vi "Matlab Param Array to Variant.vi"(8 "error in (no error)":errorcluster, 10 "Name":string, 11 "Variables":cluster{"Name":string, "Data":variant}[](array[cluster])) -> (0 "error out":errorcluster, 3 "Data":variant)   [LabVIEW 2010, in "Matlab API.lvlib"]
uses:
  Matlab API.lvlib
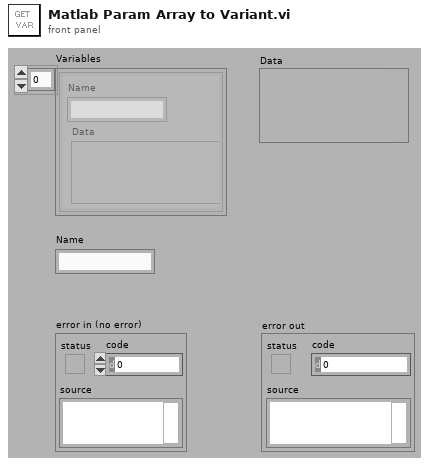
[diagram p1: front panel]
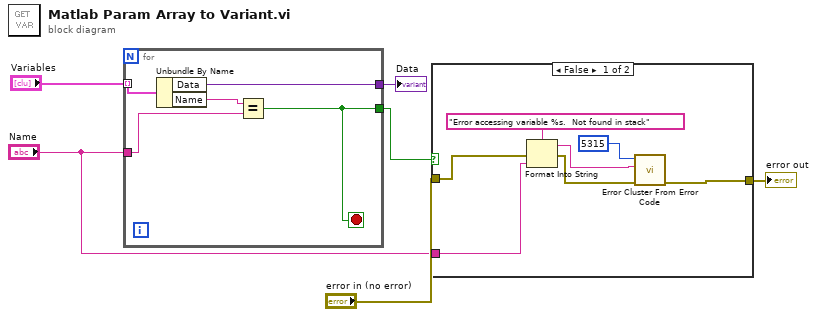
[diagram p0: block diagram]
diagram:
  n1 = for {
    tunnel: "Variables" -> [w11] mode=indexing
    tunnel: "Name" -> [w9]
    tunnel: [w8] -> w5
    tunnel: [w7] -> w1
    stop <- w8 stop-if-true
    n2 = Unbundle By Name(w11) -> ("Data"=w7:variant, "Name"=w10:string)
    n3 = Equal?(x=w10, y=w9) -> (x = y?=w8:bool)
  }
  "Data" <- w1
  n4 = case shown="False" w5 {
    tunnel: "error in (no error)" -> [w15 w19]
    tunnel: [w17 w19] -> w2
    tunnel: "Name" -> [w13 _]
    frame False {
      n5 = Format Into String(format string="Error accessing variable %s.  Not found in stack", error in=w15, w13) -> (resulting string=w12:string, error out=w14:errorcluster)  [unwired: 1 in]
      n6 = call <vilib>:"Error Cluster From Error Code.vi"("error in (no error)"=w14, "error message (\"\")"=w12, "error code (0)"=5315) -> ("error out"=w17:errorcluster)  [unwired: 1 in, 5 out]
    }
    frame True {
    }
  }
  "error out" <- w2
